vi "FTP_CreateRemotePath.vi"(5 "password":string, 7 "user":string="anonymous", 8 "error in":errorcluster, 10 "File Path":path, 11 "IP Address":string) -> (0 "error out":errorcluster)   [LabVIEW 2014, in "hse-network.lvlib"]
doc: "____\nHAMPEL SOFTWARE ENGINEERING v0.7.0 (2018-07-16 18:12)"
uses:
  hse-network.lvlib
  <vilib>/FTP/NI_FTP.lvlib
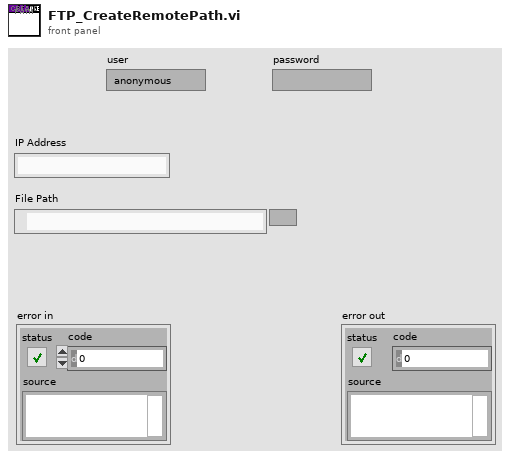
[diagram p1: front panel]
types:
  T1 = typedef "NI_FTP.lvlib/FTP Session.ctl" = refnum<k5>
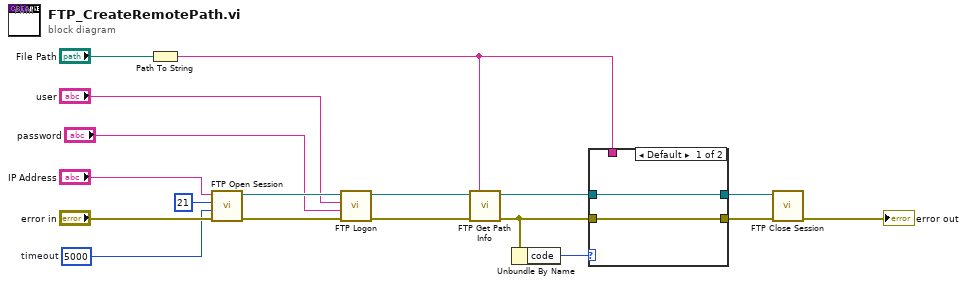
[diagram p0: block diagram]
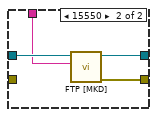
[diagram p2: hidden frame]
diagram:
  w1 = 5000  # timeout
  n1 = Path To String(path="File Path") -> (string=w4:string)
  n2 = call <vilib>:"FTP Open Session.vi"("error in (no error)"="error in", "timeout ms (60000)"=w1, "remote port (21)"=u16 21, "address"="IP Address") -> ("error out"=w13:errorcluster, "ftp session"=w12:T1)  [unwired: 4 in, 2 out]
  n3 = call <vilib>:"FTP Logon.vi"("error in (no error)"=w13, "password"="password", "user"="user", "ftp session"=w12) -> ("error out"=w10:errorcluster, "ftp session out"=w11:T1)  [unwired: 4 in, 2 out]
  n4 = call <vilib>:"FTP Get Path Info.vi"("error in (no error)"=w10, "remote path"=w4, "ftp session"=w11) -> ("error out"=w2:errorcluster, "ftp session out"=w6:T1)  [unwired: 4 in, 3 out]
  n5 = Unbundle By Name(w2) -> ("code"=w3:i32)
  n6 = case shown="Default" w3 {
    tunnel: w2 -> [w19 _]
    tunnel: [w19 w24] -> w7
    tunnel: w6 -> [w20 w23]
    tunnel: [w20 w22] -> w5
    tunnel: w4 -> [_ w21]
    frame Default {
    }
    frame 15550 {
      n7 = call <vilib>:"FTP [MKD].vi"("directory path"=w21, "ftp session"=w23) -> ("error out"=w24:errorcluster, "ftp session out"=w22:T1)  [unwired: 6 in, 2 out]
    }
  }
  n8 = call <vilib>:"FTP Close Session.vi"("error in (no error)"=w7, "ftp session"=w5) -> ("error out"=→"error out":errorcluster)  [unwired: 6 in, 3 out]
